vi "RemoteControl.STM.TestLauncher.vi"() -> ()   [LabVIEW 2016, in "RemoteControl.STM.lvclass"]
uses:
  RemoteControl.STM.lvclass
  <vilib>/JKI/JKI SMO/SMO/SMO.lvclass
  <vilib>/JKI/JKI SMO/SMO/Typedefs/SMOState --Enum.ctl
  <vilib>/NI/STM/SubVIs/MetaDataElement.ctl
  <vilib>/NI/STM/NI STM.lvlib
  C:/user/patrick/hg/levylab_util_remote/src/SMOs/RemoteControl/RemoteControl.lvclass
  C:/Program Files (x86)/National Instruments/LabVIEW 2016/vi.lib/JKI/JKI SMO/SMO/SMO.lvclass
  RemoteControl/RemoteControl.lvclass
  RemoteControl/Typedefs/PrivateEvents--RemoteControl.Configure.ctl
panel:
  out "SMO State":T1
  out "error out":errorcluster
  in  "Stop":bool
  # "RemoteControl.STM SMO Test Launcher"
  # "For instructions on how to use the JKI State Machine Objects, examples and video tutorials, visit:\nhttp://jki.net/state-machine-objects/\n\nJKI State Machine Objects™\nhttp://jki.net/state-machine-objects/\nCopyright (C) 2005-2015, JKI <info@jki.net>\nALL RIGHTS RESERVED"
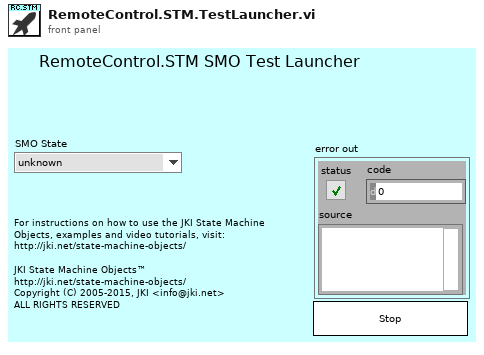
[diagram p1: front panel]
types:
  T1 = typedef "SMO.lvclass/SMOState --Enum.ctl" = enum16{"unknown", "Created", "Started", "Stopped"}
  T2 = typedef "RemoteControl.lvclass/PrivateEvents--RemoteControl.Configure.ctl" = cluster{"address":string, "Port":u32, "AllowedRemote":string, "Commands":string[]}
  T3 = typedef "NI STM.lvlib/MetaDataElement.ctl" = string
  T4 = typedef "SMO.lvclass/Public Events.ctl" = cluster{"Error":refnum<user-event>, "State":refnum<user-event>, "Reserve State":refnum<user-event>}
  T5 = cluster{"Event Registration Refnum":refnum<event-registration>}
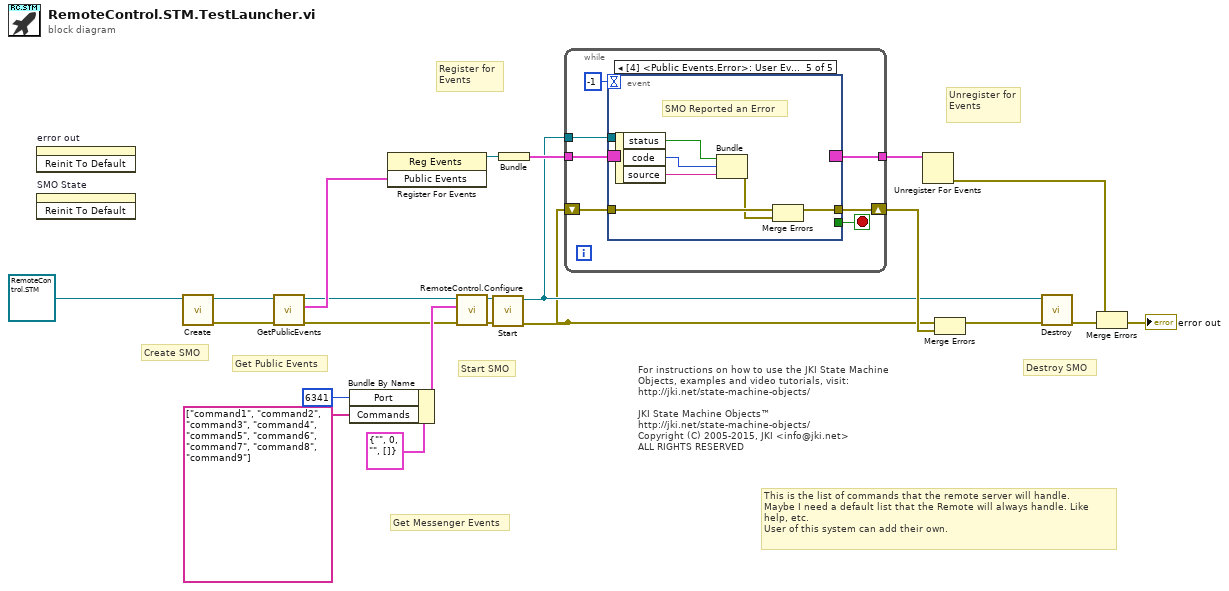
[diagram p0: block diagram]
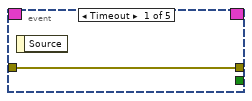
[diagram p2: hidden frame]
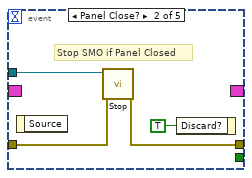
[diagram p3: hidden frame]
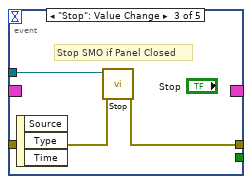
[diagram p4: hidden frame]
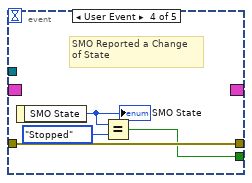
[diagram p5: hidden frame]
diagram:
  # "Get Messenger Events"
  # "This is the list of commands that the remote server will handle.\nMaybe I need a default list that the Remote will always handle. Like\nhelp, etc.\nUser of this system can add their own."
  # "For instructions on how to use the JKI State Machine Objects, examples and video tutorials, visit:\nhttp://jki.net/state-machine-objects/\n\nJKI State Machine Objects™\nhttp://jki.net/state-machine-objects/\nCopyright (C) 2005-2015, JKI <info@jki.net>\nALL RIGHTS RESERVED"
  # "Get Public Events"
  # "Start SMO"
  # "Destroy SMO"
  # "Create SMO"
  # "Unregister for Events"
  # "Register for Events"
  n1 = invoke on="error out" class="Clust (strict)" method="Reinit To Default"() -> ()  [unwired: 3 in, 3 out]
  n2 = invoke on="SMO State" class="Enum (strict)" method="Reinit To Default"() -> ()  [unwired: 3 in, 3 out]
  n3 = call <vilib>:"Create.vi"("SMO"=refnum<class "RemoteControl.STM.lvclass"> refnum ("SMO.Template.lvclass")) -> ("error out"=w13:errorcluster, "SMO out"=w12:refnum<class "RemoteControl.STM.lvclass">)  [unwired: 8 in, 1 out]
  n4 = call <vilib>:"GetPublicEvents.vi"("error in (no error)"=w13, "SMO"=w12) -> ("error out"=w6:errorcluster, "Public Events"=w15:T4, "SMO out"=w3:refnum<class "RemoteControl.STM.lvclass">)  [unwired: 7 in]
  n5 = Bundle By Name(cluster=T2 {"address"="", "Port"=0, "AllowedRemote"="", "Commands"=[]} ("Configure"), "Port"=u16 6341 ("port"), "Commands"=T3[] ["command1", "command2", "command3", "command4", "command5", "command6", "command7", "command8", "command9"] ("meta data")) -> (w8:T2)
  n6 = register-events(w15) -> (reference out=w14:refnum<event-registration>)  [unwired: 2 in, 1 out]
  n7 = call "RemoteControl.Configure.vi"("error in (no error)"=w6, "Configure"=w8, "RemoteControl"=w3) -> ("error out"=w5:errorcluster, "RemoteControl out"=w4:refnum<class "RemoteControl.STM.lvclass">)  [unwired: 7 in]
  n8 = call <vilib>:"Start.vi"("error in (no error)"=w5, "SMO"=w4) -> ("error out"=w1:errorcluster, "SMO out"=w2:refnum<class "RemoteControl.STM.lvclass">)  [unwired: 8 in]
  n9 = Bundle("Event Registration Refnum"=w14) -> (w21:T5)  [unwired: 1 in]
  n10 = while {
    shift-right: [w28] -> w20
    shift-left: w1 -> [w27]
    tunnel: w21 -> [w26]
    tunnel: [w25] -> w22
    tunnel: w2 -> [w24]
    stop <- w29 stop-if-true
    n11 = event shown="[4] <Public Events.Error>: User Event" {
      selector: w26 -> [_ _ _ _ _]
      dyn-events: [_ _ _ _ _] -> w25
      timeout: -1 -> [_ _ _ _ _]
      tunnel: [_ _ _ w38 _] -> w29
      tunnel: w24 -> [_ w34 w37 _ _]
      tunnel: [w30 w33 w36 w41 w45] -> w28
      tunnel: w27 -> [w30 w32 w35 w41 w43]
      event Timeout {
        n12 = event-data() -> ()  [unwired: 1 in, 1 out]
      }
      event Panel Close? {
        # "Stop SMO if Panel Closed"
        n13 = event-data() -> ()  [unwired: 1 in, 1 out]
        n14 = call <vilib>:"Stop.vi"("error in (no error)"=w32, "SMO"=w34) -> ("error out"=w33:errorcluster)  [unwired: 8 in, 1 out]
        n15 = event-data("Discard?"=TRUE ("OK")) -> ()  [unwired: 1 in, 1 out]
      }
      event "Stop": Value Change {
        # "Stop SMO if Panel Closed"
        n16 = event-data() -> ()  [unwired: 1 in, 3 out]
        n17 = call <vilib>:"Stop.vi"("error in (no error)"=w35, "SMO"=w37) -> ("error out"=w36:errorcluster)  [unwired: 8 in, 1 out]
      }
      event User Event {
        # "SMO Reported a Change\nof State"
        n18 = event-data() -> ("SMO State"=w40:T1)  [unwired: 1 in]
        "SMO State" <- w40
        n19 = Equal?(x=w40, y=SMOState_--Enum."Stopped") -> (x = y?=w38:bool)
      }
      event User Event {
        # "SMO Reported an Error"
        n20 = event-data() -> ("status"=w44:bool, "code"=w47:i32, "source"=w46:string)  [unwired: 1 in]
        n21 = Bundle("status"=w44, "code"=w47, "source"=w46) -> (w42:errorcluster)  [unwired: 1 in]
        n22 = Merge Errors(w43, w42) -> (w45:errorcluster)
      }
    }
  }
  n23 = Unregister For Events(event registration refnum=w22) -> (error out=w19:errorcluster)  [unwired: 1 in]
  n24 = Merge Errors(w1, w20) -> (w16:errorcluster)
  n25 = call <vilib>:"Destroy.vi"("error in (no error)"=w16, "SMO"=w2) -> ("error out"=w17:errorcluster)  [unwired: 9 in]
  n26 = Merge Errors(w19, w17) -> (→"error out":errorcluster)
